vi "Vision.vi"(0 "Image In":T3(plugin-control), 5 "Hue Range":cluster{"Lower value":i32, "Upper value":i32}={"Lower value"=0, "Upper value"=255}, 7 "Sat Range":cluster{"Lower value":i32, "Upper value":i32}={"Lower value"=0, "Upper value"=255}, 9 "Luma Range":cluster{"Lower value":i32, "Upper value":i32}={"Lower value"=0, "Upper value"=255}) -> (1 "Particle Out Paired":T3(plugin-control), 2 "Particle Out":T3(plugin-control), 3 "Thresholded Out":T3(plugin-control), 4 "Final Out":T3(plugin-control), 14 "Out":T2)   [LabVIEW 2016]
uses:
  <vilib>/vision/NI_Vision_Development_Module.lvlib
panel:
  in  "Origin":cluster{"X":i32, "Y":i32}
  in  "Font":T1={"Desired Font (Application)"=enum."Application Font", "[User-specified Font]"={"Font Name"="", "Size"=12, "Strikeout?"=FALSE, "Italic?"=FALSE, "Underline?"=FALSE, "Outline?"=FALSE, "Shadow?"=FALSE, "Bold?"=FALSE, "Rotation Angle"=0.0}, "Horizontal Alignment"=0, "Vertical Alignment"=0} {"Horizontal Alignment" items=["Left", "Center", "Right"]; "Vertical Alignment" items=["Bottom", "Top", "Baseline"]}
  in  "Default":T2
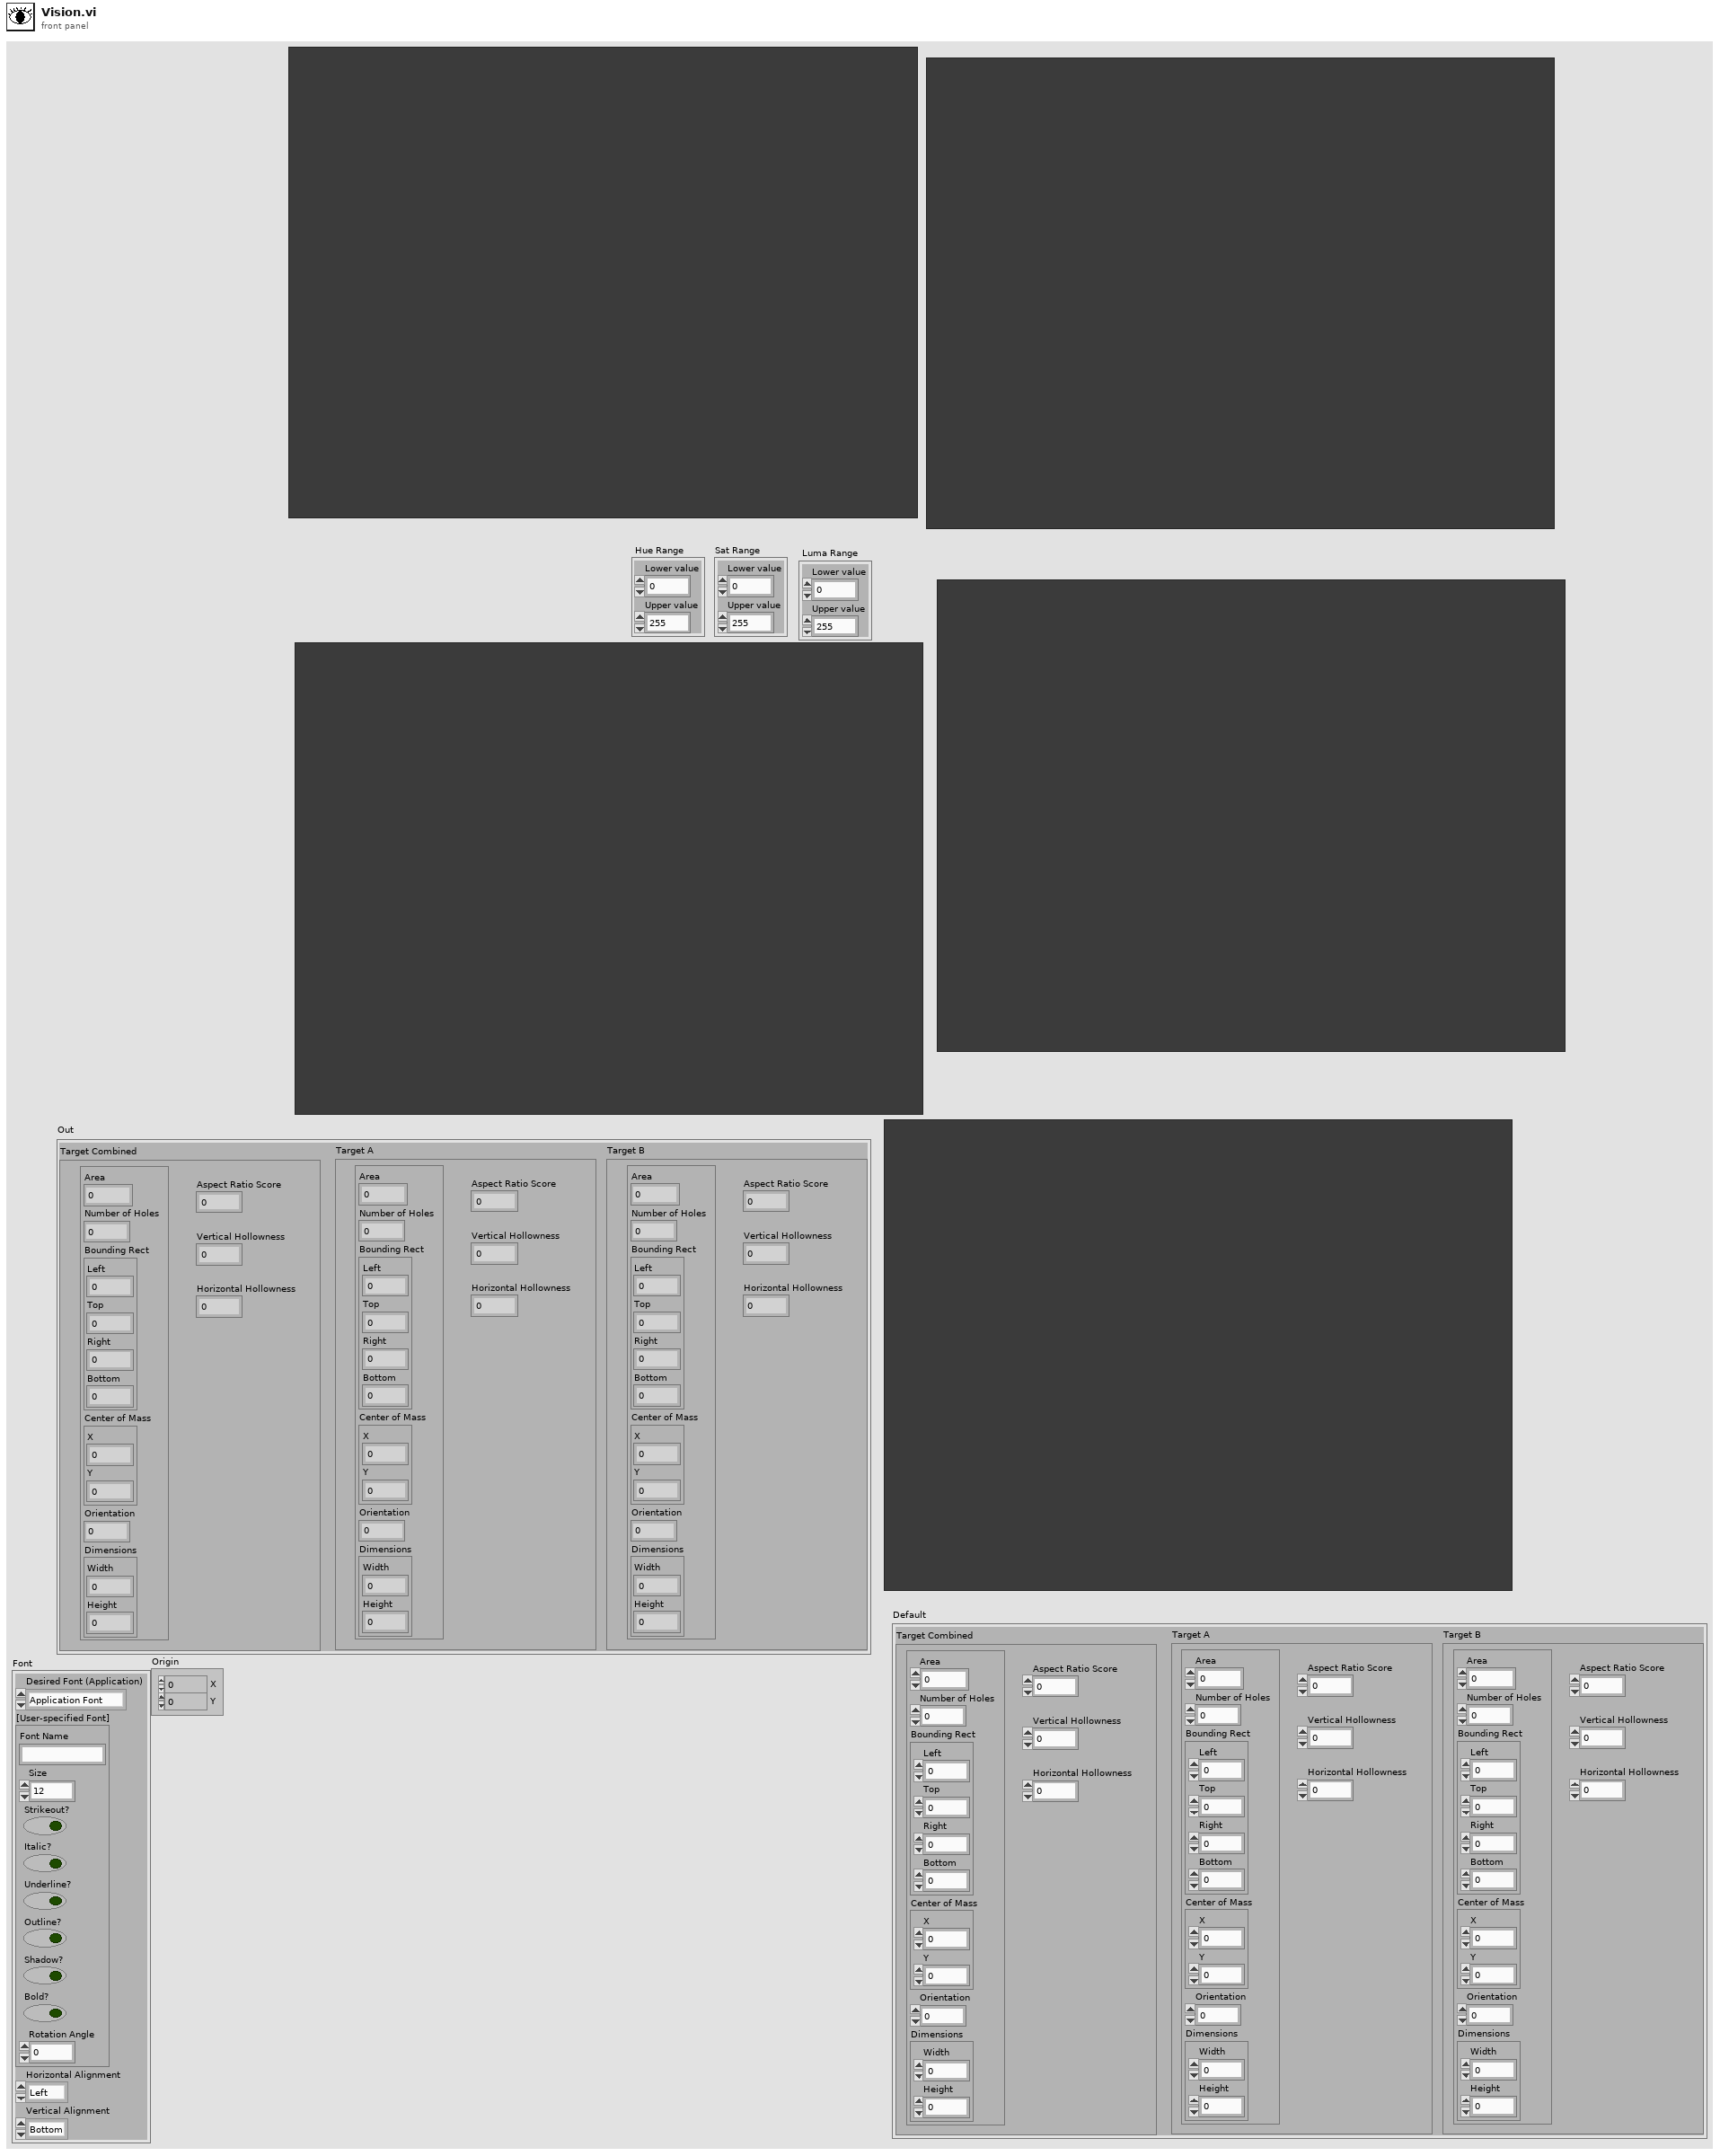
[diagram p1: front panel]
types:
  T1 = cluster{"Desired Font (Application)":enum16{"User-specified Font", "Application Font", "System Font", "Dialog Font"}, "[User-specified Font]":cluster{"Font Name":string, "Size":i16, "Strikeout?":bool, "Italic?":bool, "Underline?":bool, "Outline?":bool, "Shadow?":bool, "Bold?":bool, "Rotation Angle":dbl}, "Horizontal Alignment":i16, "Vertical Alignment":i16}
  T2 = cluster{"Target Combined":cluster{"Particle Report":cluster{"Area":dbl, "Number of Holes":dbl, "Bounding Rect":cluster{"Left":dbl, "Top":dbl, "Right":dbl, "Bottom":dbl}, "Center of Mass":cluster{"X":dbl, "Y":dbl}, "Orientation":dbl, "Dimensions":cluster{"Width":dbl, "Height":dbl}}, "Aspect Ratio Score":dbl, "Vertical Hollowness":dbl, "Horizontal Hollowness":dbl}, "Target A":cluster{"Particle Report":cluster{"Area":dbl, "Number of Holes":dbl, "Bounding Rect":cluster{"Left":dbl, "Top":dbl, "Right":dbl, "Bottom":dbl}, "Center of Mass":cluster{"X":dbl, "Y":dbl}, "Orientation":dbl, "Dimensions":cluster{"Width":dbl, "Height":dbl}}, "Aspect Ratio Score":dbl, "Vertical Hollowness":dbl, "Horizontal Hollowness":dbl}, "Target B":cluster{"Particle Report":cluster{"Area":dbl, "Number of Holes":dbl, "Bounding Rect":cluster{"Left":dbl, "Top":dbl, "Right":dbl, "Bottom":dbl}, "Center of Mass":cluster{"X":dbl, "Y":dbl}, "Orientation":dbl, "Dimensions":cluster{"Width":dbl, "Height":dbl}}, "Aspect Ratio Score":dbl, "Vertical Hollowness":dbl, "Horizontal Hollowness":dbl}}
  T3 = typedef "IMAQ Image.ctl" = refnum<image>
  T4 = cluster{"Area":dbl, "Number of Holes":dbl, "Bounding Rect":cluster{"Left":dbl, "Top":dbl, "Right":dbl, "Bottom":dbl}, "Center of Mass":cluster{"X":dbl, "Y":dbl}, "Orientation":dbl, "Dimensions":cluster{"Width":dbl, "Height":dbl}}[]
  T5 = typedef "Image Type" = u32
  T6 = cluster{"Particle Report":cluster{"Area":dbl, "Number of Holes":dbl, "Bounding Rect":cluster{"Left":dbl, "Top":dbl, "Right":dbl, "Bottom":dbl}, "Center of Mass":cluster{"X":dbl, "Y":dbl}, "Orientation":dbl, "Dimensions":cluster{"Width":dbl, "Height":dbl}}, "Aspect Ratio Score":dbl, "Vertical Hollowness":dbl, "Horizontal Hollowness":dbl}
  T7 = cluster{"Target Combined":cluster{"Particle Report":cluster{"Area":dbl, "Number of Holes":dbl, "Bounding Rect":cluster{"Left":dbl, "Top":dbl, "Right":dbl, "Bottom":dbl}, "Center of Mass":cluster{"X":dbl, "Y":dbl}, "Orientation":dbl, "Dimensions":cluster{"Width":dbl, "Height":dbl}}, "Aspect Ratio Score":dbl, "Vertical Hollowness":dbl, "Horizontal Hollowness":dbl}, "Target A":cluster{"Particle Report":cluster{"Area":dbl, "Number of Holes":dbl, "Bounding Rect":cluster{"Left":dbl, "Top":dbl, "Right":dbl, "Bottom":dbl}, "Center of Mass":cluster{"X":dbl, "Y":dbl}, "Orientation":dbl, "Dimensions":cluster{"Width":dbl, "Height":dbl}}, "Aspect Ratio Score":dbl, "Vertical Hollowness":dbl, "Horizontal Hollowness":dbl}, "Target B":cluster{"Particle Report":cluster{"Area":dbl, "Number of Holes":dbl, "Bounding Rect":cluster{"Left":dbl, "Top":dbl, "Right":dbl, "Bottom":dbl}, "Center of Mass":cluster{"X":dbl, "Y":dbl}, "Orientation":dbl, "Dimensions":cluster{"Width":dbl, "Height":dbl}}, "Aspect Ratio Score":dbl, "Vertical Hollowness":dbl, "Horizontal Hollowness":dbl}}[]
  T8 = cluster{"Left":dbl, "Top":dbl, "Right":dbl, "Bottom":dbl}
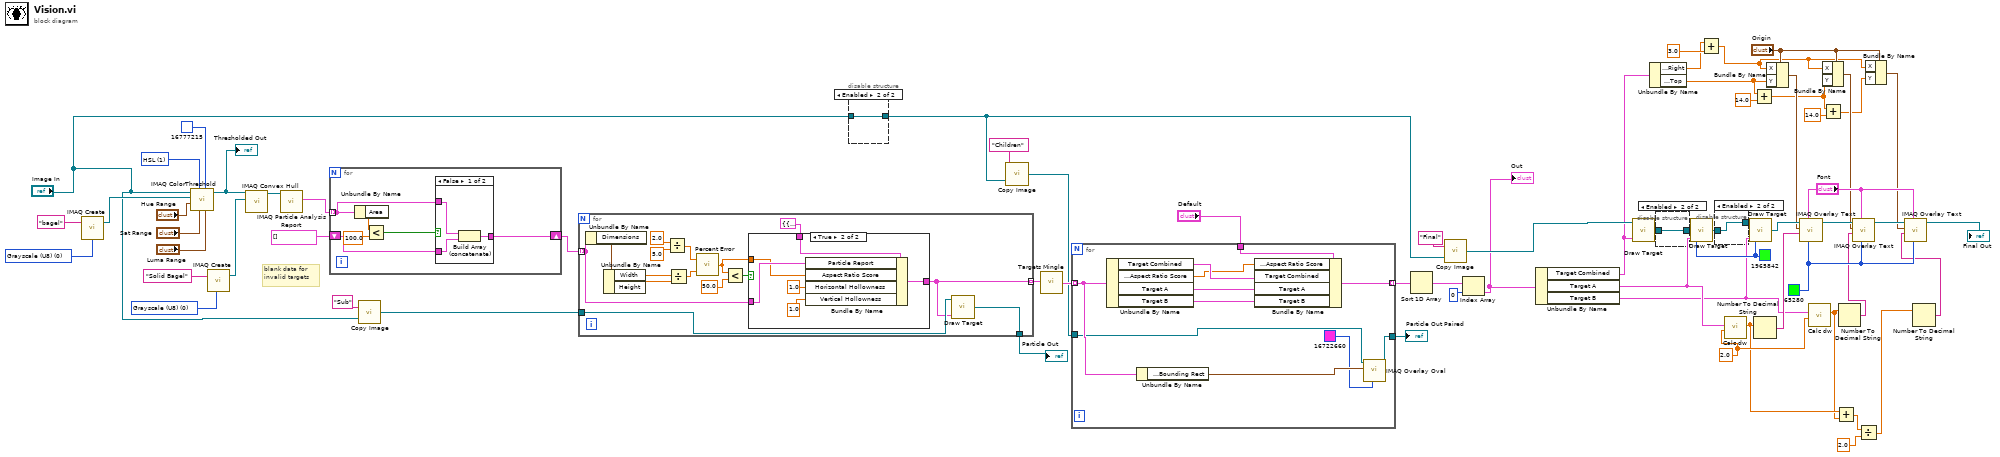
[diagram p0: block diagram]
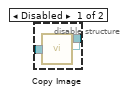
[diagram p2: hidden frame]
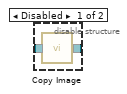
[diagram p3: hidden frame]
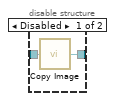
[diagram p4: hidden frame]
diagram:
  w23 = 2.0
  w28 = u32 65280 ("Color Box")
  w37 = u32 1965842 ("Color Box")
  w49 = u16 1 items=["RGB", "HSL", "HSV", "HSI"] ("Color Mode")
  w62 = T5 0 items=["Grayscale (U8)", "Grayscale (I16)", "Grayscale (SGL)", "Complex (CSG)", "RGB (U32)", "HSL (U32)", "RGB (U64)", "Grayscale (U16)"] ("Image Type")
  w64 = T5 0 items=["Grayscale (U8)", "Grayscale (I16)", "Grayscale (SGL)", "Complex (CSG)", "RGB (U32)", "HSL (U32)", "RGB (U64)", "Grayscale (U16)"] ("Image Type")
  # "blank data for \ninvalid targets"
  n1 = call "IMAQ Create"("Image Name"="bagel", "Image Type"=w64) -> ("New Image"=w63:T3)  [unwired: 3 in, 1 out]
  n2 = call "IMAQ ColorThreshold"("Blue or Luma or Val or Inten Range"="Luma Range", "Replace Value"=u32 16777215 ("Color Box"), "Green or Sat Range"="Sat Range", "Color Mode"=w49, "Red or Hue Range"="Hue Range", "Image Dst"=w63, "Image Src"="Image In") -> ("Image Dst Out"=w50:T3)  [unwired: 3 in, 1 out]
  "Thresholded Out" <- w50
  n3 = call "IMAQ Create"("Image Name"="Solid Bagel", "Image Type"=w62) -> ("New Image"=w61:T3)  [unwired: 3 in, 1 out]
  n4 = call "IMAQ Convex Hull"("Image Dst"=w61, "Image Src"=w50) -> ("Image Dst Out"=w47:T3)  [unwired: 8 in, 1 out]
  n5 = call "IMAQ Particle Analysis Report"("Image"=w47) -> ("Particle Reports (Pixels)"=w59:T4)  [unwired: 5 in, 5 out]
  n6 = for {
    tunnel: w59 -> [w71] mode=indexing
    shift-right: [w70] -> w58
    shift-left: T4 [] -> [w69]
    n7 = Unbundle By Name(w71) -> ("Area"=w74:dbl)
    n8 = Less?(x=w74, y=100.0) -> (x < y?=w72:bool)
    n9 = case shown="False" w72 {
      tunnel: w71 -> [w77 _]
      tunnel: [w76 w78] -> w70
      tunnel: w69 -> [w75 w78]
      frame False {
        n10 = Build Array (concatenate)(w77, w75) -> (w76:T4)
      }
      frame True {
      }
    }
  }
  n11 = call "Copy Image.vi"("Image In"="Image In", "Name"="Sub") -> ("Image Out"=w45:T3)
  n12 = for {
    tunnel: w58 -> [w84] mode=indexing
    tunnel: [w80] -> w56 mode=indexing
    tunnel: w45 -> [w81]
    tunnel: [w79] -> w40
    n13 = Unbundle By Name(w84) -> ("Dimensions"=w93:cluster{"Width":dbl, "Height":dbl})
    n14 = Unbundle By Name(w93) -> ("Width"=w92:dbl, "Height"=w91:dbl)
    n15 = Divide(x=2.0, y=5.0) -> (x/y=w89:dbl)
    n16 = Divide(x=w92, y=w91) -> (x/y=w90:dbl)
    n17 = call "Percent Error.vi"("Measured Values"=w90, "Accepted Value"=w89) -> ("Percent Error"=w82:dbl)
    n18 = Less?(x=w82, y=50.0) -> (x < y?=w86:bool)
    n19 = case shown="True" w86 {
      tunnel: w84 -> [_ w100]
      tunnel: [w94 w99] -> w80
      tunnel: T6 {"Particle Report"={"Area"=0.0, "Number of Holes"=0.0, "Bounding Rect"={"Left"=0.0, "Top"=0.0, "Right"=0.0, "Bottom"=0.0}, "Center of Mass"={"X"=0.0, "Y"=0.0}, "Orientation"=0.0, "Dimensions"={"Width"=0.0, "Height"=0.0}}, "Aspect Ratio Score"=0.0, "Vertical Hollowness"=0.0, "Horizontal Hollowness"=0.0} ("Cluster") -> [w94 w97]
      tunnel: w82 -> [_ w98]
      frame False {
      }
      frame True {
        n20 = Bundle By Name(cluster=w97, "Particle Report"=w100, "Aspect Ratio Score"=w98, "Horizontal Hollowness"=1.0, "Vertical Hollowness"=1.0) -> (w99:T6)
      }
    }
    n21 = call "Draw Target.vi"("Cluster"=w80, "In"=w81) -> ("Out"=w79:T3)  [unwired: 1 in]
  }
  "Particle Out" <- w40
  n22 = disable-structure shown="Enabled" {
    disable-tunnel: "Image In" -> [w102 w103]
    disable-tunnel: [w101 w103] -> w42
    frame Disabled {
      n23 = call "Copy Image.vi"("Image In"=w102) -> ("Image Out"=w101:T3)
    }
    frame Enabled {
    }
  }
  n24 = call "Copy Image.vi"("Image In"=w42, "Name"="Children") -> ("Image Out"=w44:T3)
  n25 = call "Targets Mingle.vi"("Single Targets"=w56) -> ("Married Targets"=w55:T7)
  n26 = for {
    tunnel: w55 -> [w110] mode=indexing
    tunnel: "Default" -> [w114]
    tunnel: [w111] -> w53 mode=indexing
    tunnel: [w106] -> w46
    tunnel: w44 -> [w107]
    n27 = Unbundle By Name(w110) -> ("Target Combined"=w113:T6, "Target Combined.Aspect Ratio Score"=w112:dbl, "Target A"=w109:T6, "Target B"=w108:T6)
    n28 = Unbundle By Name(w110) -> ("Target Combined.Particle Report.Bounding Rect"=w105:T8)
    n29 = Bundle By Name(cluster=w114, "Target Combined.Aspect Ratio Score"=w112, "Target Combined"=w113, "Target A"=w109, "Target B"=w108) -> (w111:T2)
    n30 = call "IMAQ Overlay Oval"("Color"=u32 16722660 ("Color Box"), "Bounding Rectangle"=w105, "Image"=w107) -> ("Image Out"=w106:T3)  [unwired: 7 in, 1 out]
  }
  "Particle Out Paired" <- w46
  n31 = Sort 1D Array(array=w53) -> (sorted array=w52:T7)
  n32 = call "Copy Image.vi"("Image In"=w42, "Name"="Final") -> ("Image Out"=w41:T3)
  n33 = Index Array(array=w52, index=0) -> (element=w39:T2)
  "Out" <- w39
  n34 = Unbundle By Name(w39) -> ("Target Combined"=w20:T6, "Target A"=w31:T6, "Target B"=w24:T6)
  n35 = call "Draw Target.vi"("Cluster"=w20, "In"=w41) -> ("Out"=w36:T3)  [unwired: 1 in]
  n36 = Unbundle By Name(w20) -> ("Particle Report.Bounding Rect.Right"=w9:dbl, "Particle Report.Bounding Rect.Top"=w17:dbl)
  n37 = disable-structure shown="Enabled" {
    disable-tunnel: w36 -> [w116 w117]
    disable-tunnel: [w115 w117] -> w35
    frame Disabled {
      n38 = call "Copy Image.vi"("Image In"=w116) -> ("Image Out"=w115:T3)
    }
    frame Enabled {
    }
  }
  n39 = call "Draw Target.vi"("Cluster"=w31, "Color Box"=w37, "In"=w35) -> ("Out"=w34:T3)
  n40 = Add(x=w9, y=3.0) -> (x+y=w10:dbl)
  n41 = disable-structure shown="Enabled" {
    disable-tunnel: w34 -> [w119 w120]
    disable-tunnel: [w118 w120] -> w33
    frame Disabled {
      n42 = call "Copy Image.vi"("Image In"=w119) -> ("Image Out"=w118:T3)
    }
    frame Enabled {
    }
  }
  n43 = call "Calc dw.vi"("Width T in incheees"=w23, "Target"=w31) -> ("dw"=w6:dbl)  [unwired: 9 in]
  n44 = call "Draw Target.vi"("Cluster"=w24, "Color Box"=w37, "In"=w33) -> ("Out"=w32:T3)
  n45 = Add(x=w17, y=14.0) -> (x+y=w13:dbl)
  n46 = Number To Decimal String(number=w6) -> (decimal integer string=w30:string)  [unwired: 1 in]
  n47 = Bundle By Name(cluster="Origin", "X"=w10, "Y"=w17) -> (w21:cluster{"X":i32, "Y":i32})
  n48 = call "IMAQ Overlay Text"("Text Color (black)"=w28, "Font, Size & Style"="Font", "String"=w30, "Origin"=w21, "Image"=w32) -> ("Image Out"=w26:T3)  [unwired: 5 in, 1 out]
  n49 = call "Calc dw.vi"("Width T in incheees"=w23, "Target"=w24) -> ("dw"=w5:dbl)  [unwired: 9 in]
  n50 = Bundle By Name(cluster="Origin", "X"=w10, "Y"=w13) -> (w19:cluster{"X":i32, "Y":i32})
  n51 = Add(x=w13, y=14.0) -> (x+y=w12:dbl)
  n52 = Add(x=w6, y=w5) -> (x+y=w7:dbl)
  n53 = Number To Decimal String(number=w5) -> (decimal integer string=w27:string)  [unwired: 1 in]
  n54 = call "IMAQ Overlay Text"("Text Color (black)"=w28, "Font, Size & Style"="Font", "String"=w27, "Origin"=w19, "Image"=w26) -> ("Image Out"=w25:T3)  [unwired: 5 in, 1 out]
  n55 = Divide(x=w7, y=2.0) -> (x/y=w4:dbl)
  n56 = Bundle By Name(cluster="Origin", "X"=w10, "Y"=w12) -> (w15:cluster{"X":i32, "Y":i32})
  n57 = Number To Decimal String(number=w4) -> (decimal integer string=w22:string)  [unwired: 1 in]
  n58 = call "IMAQ Overlay Text"("Text Color (black)"=w28, "Font, Size & Style"="Font", "String"=w22, "Origin"=w15, "Image"=w25) -> ("Image Out"=→"Final Out":T3)  [unwired: 5 in, 1 out]
